vi "Day 11 Array Manipulation Engines.vi"() -> ()   [LabVIEW 2026]
panel:
  out "Column Sum":dbl
  out "Row Sum":dbl
  in  "Column Choice":i32
  in  "Row choice":i32
  in  "Array 3":dbl[][](array[numeric])
  out "min value":dbl
  out "max value":dbl
  out "reversed array":dbl[](array[numeric])
  in  "Array 2":dbl[](array[numeric])
  in  "index":i32
  out "element":dbl
  out "size(s)":i32
  in  "Array":dbl[](array[numeric])
  # "Build, index, and get the size of a 1D array"
  # "Reverse an array and find its max/min with array-palette functions"
  # "Given a 2D array, extract a specified row and column and compute their sums."
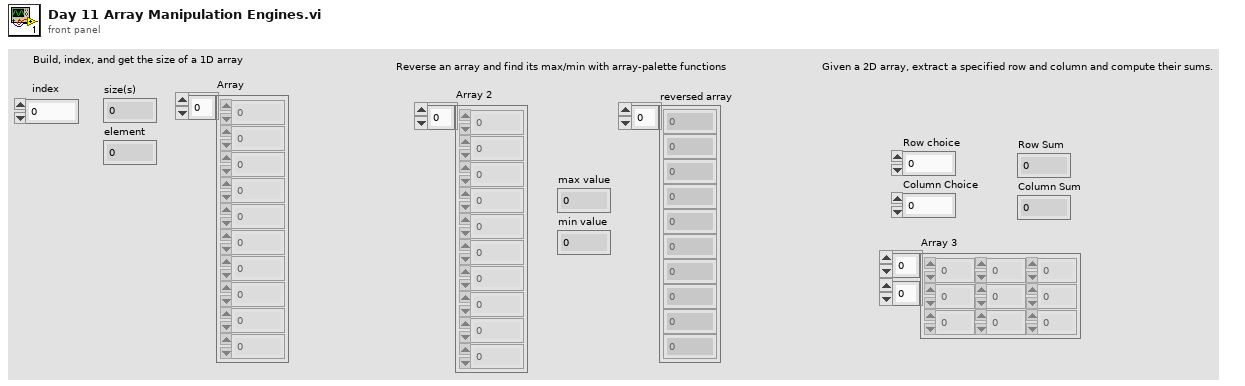
[diagram p1: front panel]
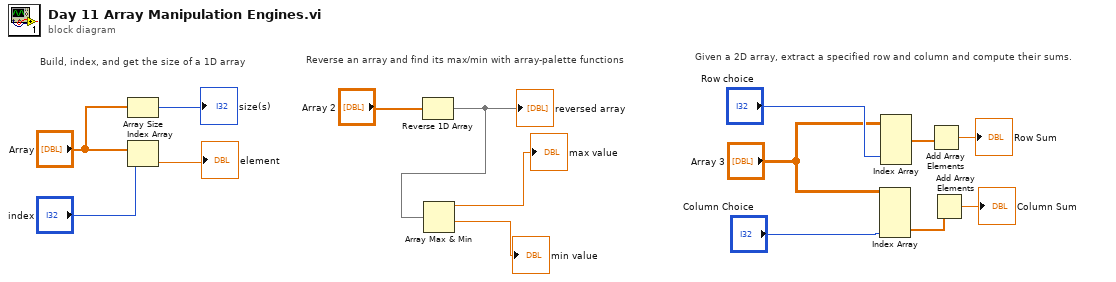
[diagram p0: block diagram]
diagram:
  # "Reverse an array and find its max/min with array-palette functions"
  # "Build, index, and get the size of a 1D array"
  # "Given a 2D array, extract a specified row and column and compute their sums."
  n1 = Array Size(array="Array") -> (size(s)=→"size(s)":i32)
  n2 = Index Array "Index Array"(array="Array", index="index") -> (element=→"element":dbl)
  n3 = Reverse 1D Array(array="Array 2") -> (reversed array=w10:dbl[])
  "reversed array" <- w10
  n4 = Array Max & Min(array=w10) -> (max value=→"max value":dbl, min value=→"min value":dbl)  [unwired: 2 out]
  n5 = Index Array(array="Array 3", index (col) #2="Column Choice") -> (element #2=w2:dbl[])  [unwired: 3 in, 1 out]
  n6 = Index Array(array="Array 3", index (row) #1="Row choice") -> (element #1=w3:dbl[])  [unwired: 3 in, 1 out]
  n7 = Add Array Elements(numeric array=w3) -> (sum=→"Row Sum":dbl)
  n8 = Add Array Elements(numeric array=w2) -> (sum=→"Column Sum":dbl)
